vi "sub_trigger-check3.vi"(7 "cmd":enum16{"check", "clear"}(ring), 11 "log data":T1={"strain filter_n_nulling wf"=[], "force wf"={"t0"=timestamp(0 s since 1904-01-01), "dt"=1.0, "Y"=[]}, "force"=-260.0, "Balance xy wfs"=[{"X"=-0.16459892377479407, "Y"=-3.796401322594745}, {"X"=0.01591661701557069, "Y"=-0.7378646010803016}, {"X"=0.008943048340024115, "Y"=-0.649392437584039}, {"X"=0.07222606467199857, "Y"=0.7586688854530768}], "vacuum kpa wf"={"t0"=timestamp(0 s since 1904-01-01), "dt"=1.0, "Y"=[]}, "pcb temp"=[]}) -> (3 "trigger":bool)   [LabVIEW 2016]
uses:
  ctl/log_data.ctl
  <vilib>/Analysis/baseanly.llb/Mean (DBL).vi
  <vilib>/Analysis/NI_AALBase.lvlib
panel:
  out "웨이브폼 차트":cluster{"vacuum":dbl, "force":dbl}(graph)
  out "cnt":i32
  out "출력 클러스터":cluster{"Value":dbl, "force_cal":dbl}
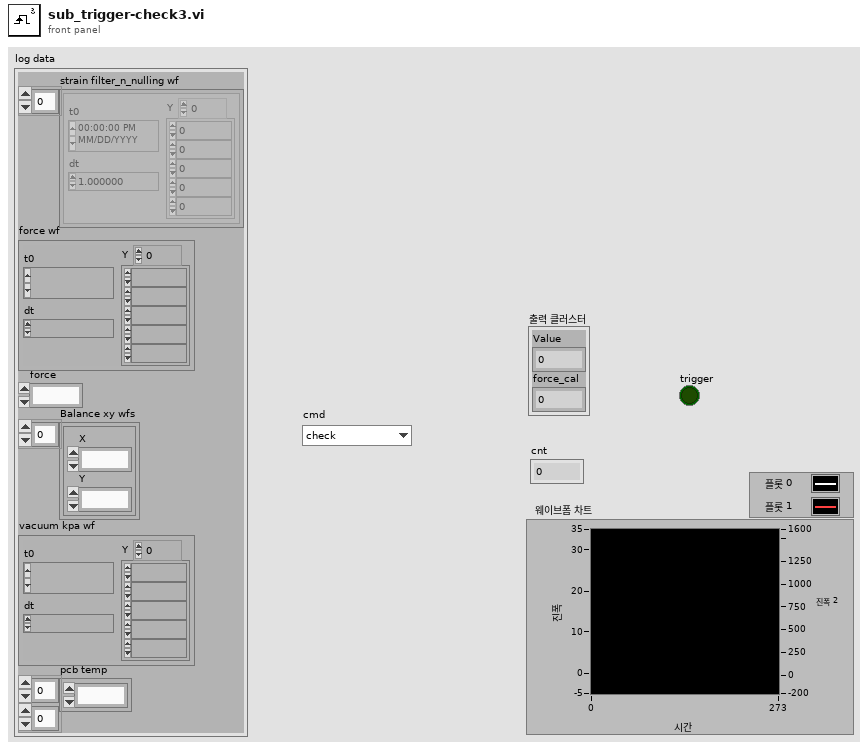
[diagram p1: front panel]
types:
  T1 = typedef "log_data.ctl" = cluster{"strain filter_n_nulling wf":waveform(dbl)[], "force wf":waveform(dbl), "force":dbl, "Balance xy wfs":cluster{"X":dbl, "Y":dbl}[], "vacuum kpa wf":waveform(dbl), "pcb temp":dbl[][]}
  T2 = typedef "config_ctl.ctl" = cluster{"Lower Cut-Off":dbl, "Vacuum Trigger level":dbl, "state settings":cluster{"method":enum32{"histogram", "peak", "auto select"}, "histogram size":i32, "histogram method":enum16{"mode"}, "reserved":dbl}, "SPA-300 Setting":cluster{"Bonding force (g)":dbl, "Bonding time (ms)":dbl, "Pickup force (g)":dbl, "Pickup time (ms)":dbl, "Speed":enum16{"Slow", "Fast"}}, "sensor file":path}
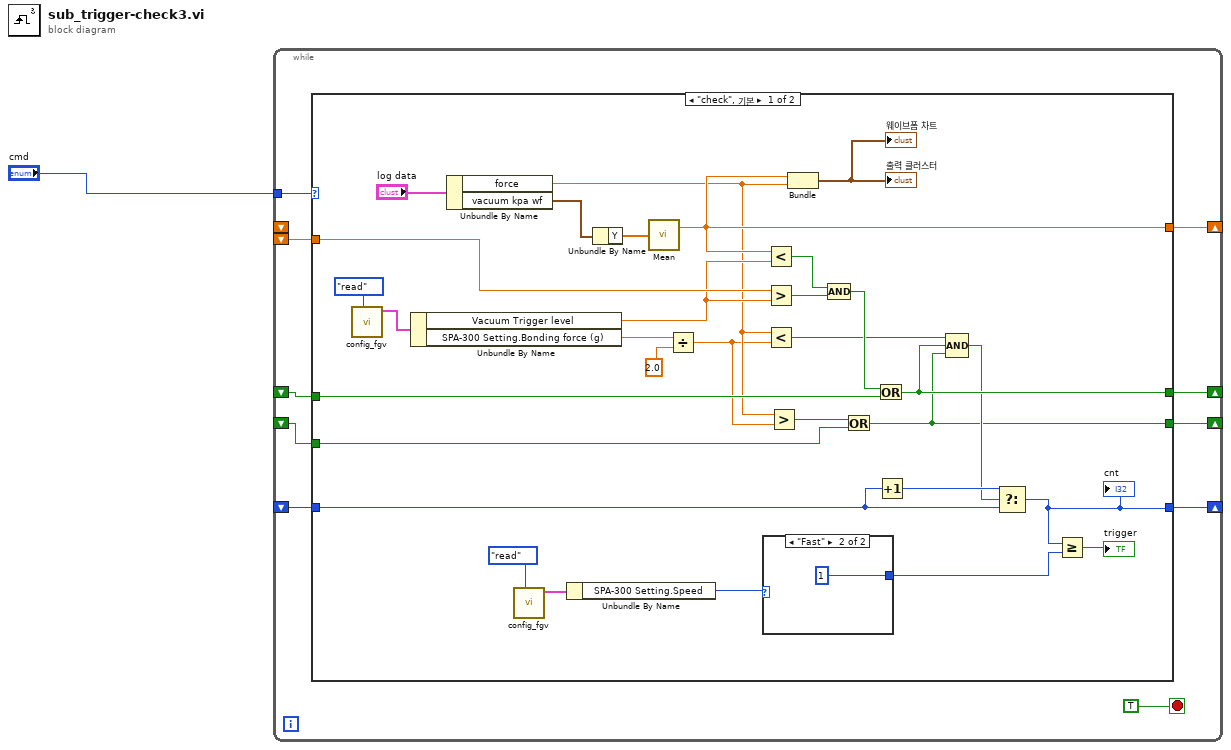
[diagram p0: block diagram]
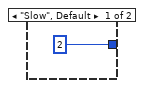
[diagram p2: hidden frame]
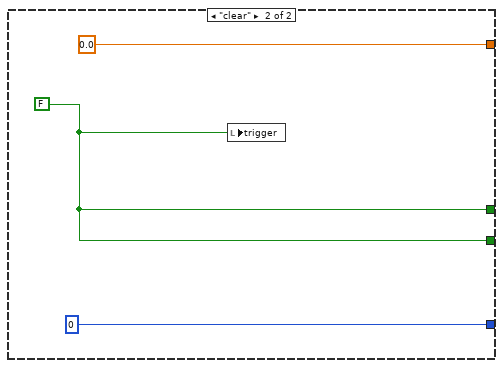
[diagram p3: hidden frame]
diagram:
  n1 = while {
    tunnel: "cmd" -> [w10]
    shift-right: [w9] -> _
    shift-left: _ -> [_]
    shift-left: _ -> [w4]
    shift-right: [w8] -> _
    shift-left: _ -> [w5]
    shift-right: [w7] -> _
    shift-left: _ -> [w6]
    shift-right: [w2] -> _
    shift-left: _ -> [w3]
    stop <- TRUE stop-if-true
    n2 = case shown="\"check\", 기본" w10 {
      tunnel: [w23 0.0] -> w9
      tunnel: [w36 0] -> w8
      tunnel: [w28 w45] -> w7
      tunnel: w6 -> [w40 _]
      tunnel: w5 -> [w38 _]
      tunnel: w4 -> [w35 _]
      tunnel: w3 -> [w17 _]
      tunnel: [w16 w45] -> w2
      frame "check", Default {
        n3 = call "config_fgv.vi"("cmd"=enum16{"write", "read", "ini"}."read") -> ("Config out"=w33:T2)  [unwired: 9 in, 1 out]
        n4 = Unbundle By Name(w33) -> ("Vacuum Trigger level"=w32:dbl, "SPA-300 Setting.Bonding force (g)"=w30:dbl)
        n5 = Unbundle By Name("log data") -> ("force"=w20:dbl, "vacuum kpa wf"=w21:waveform(dbl))
        n6 = call "config_fgv.vi"("cmd"=enum16{"write", "read", "ini"}."read") -> ("Config out"=w14:T2)  [unwired: 9 in, 1 out]
        n7 = Unbundle By Name(w14) -> ("SPA-300 Setting.Speed"=w13:enum16{"Slow", "Fast"})
        n8 = Unbundle By Name(w21) -> ("Y"=w24:dbl[])
        n9 = call-poly <vilib>:"Mean.vi"("X"=w24) -> ("mean"=w23:dbl)  [unwired: 1 out]
        n10 = Divide(x=w30, y=2.0) -> (x/y=w19:dbl)
        n11 = case shown="\"Fast\"" w13 {
          tunnel: [2 ("count") 1 ("count")] -> w12
          frame "Slow", Default {
          }
          frame "Fast" {
          }
        }
        n12 = Less?(x=w23, y=w32) -> (x < y?=w41:bool)
        n13 = Greater?(x=w35, y=w32) -> (0:w42:bool)
        n14 = Less?(x=w20, y=w19) -> (x < y?=w26:bool)
        n15 = Greater?(x=w20, y=w19) -> (0:w18:bool)
        n16 = Bundle("mean"=w23, "force"=w20) -> (→"출력 클러스터" →"웨이브폼 차트":cluster{"mean":dbl, "force":dbl})  [unwired: 1 in]
        n17 = Compound Arithmetic op=AND(w41, w42) -> (w27:bool)
        n18 = Or(x=w18, y=w17) -> (x .or. y?=w16:bool)
        n19 = Or(x=w27, y=w40) -> (x .or. y?=w28:bool)
        n20 = Increment(x=w38) -> (x+1=w39:i32)
        n21 = Compound Arithmetic op=AND(w26, w28, w16) -> (w25:bool)
        n22 = Select(t=w39, s=w25, f=w38) -> (s? t:f=w36:i32)
        "cnt" <- w36
        n23 = Greater Or Equal?(x=w36, y=w12) -> (x >= y?=→"trigger":bool)
      }
      frame "clear" {
        w45 = FALSE
        n24 = local write "trigger"(w45) -> ()
      }
    }
  }
